vi "RED.vi"(1 "Value In":bool) -> (0 "Rising Edge":bool)   [LabVIEW 2014]
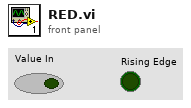
[diagram p1: front panel]
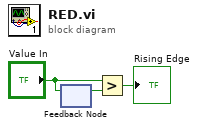
[diagram p0: block diagram]
diagram:
  n1 = feedback-in #1("Value In") -> ()
  n2 = feedback #1() -> (w2:bool)  [unwired: 1 in]
  n3 = Greater?(x="Value In", y=w2) -> (0:→"Rising Edge":bool)
